vi "Find Monitor Recorders.vi"(8 "error in (no error)":errorcluster, 11 "Monitor-Pulse in":refnum<class "Monitor-Pulse.lvclass">) -> (0 "error out":errorcluster, 2 "Actot names out":string[](array[string]), 3 "Monitor-Pulse out":refnum<class "Monitor-Pulse.lvclass">)   [LabVIEW 2015, in "Monitor-Pulse.lvclass"]
uses:
  Monitor-Pulse.lvclass
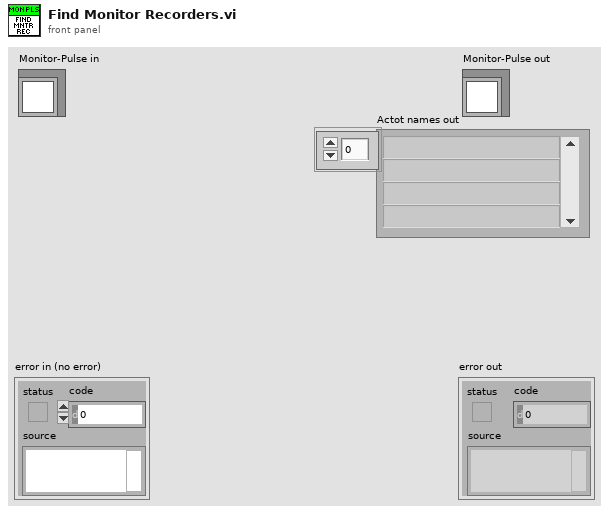
[diagram p1: front panel]
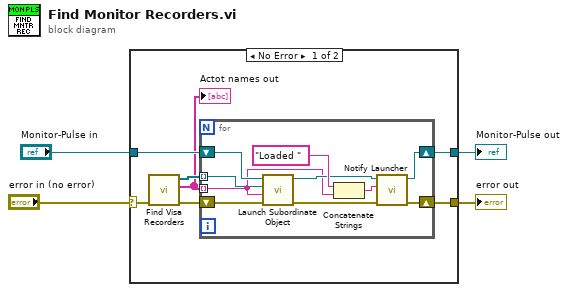
[diagram p0: block diagram]
diagram:
  n1 = case shown="No Error" "error in (no error)" {
    selector: "error in (no error)" -> [w11 w23]
    tunnel: [w7 w23] -> w3
    tunnel: [w9 w22] -> w1
    tunnel: "Monitor-Pulse in" -> [w10 w22]
    frame No Error {
      n2 = call "Find Visa Recorders.vi"("Error In"=w11) -> ("Error Out"=w8:errorcluster, "Names"=w5:string[], "Recorders List"=w6:refnum<class "Instrument Recorder.lvclass">[])  [unwired: 8 in]
      "Actot names out" <- w5
      n3 = for {
        shift-right: [w15] -> w9
        shift-left: w10 -> [w21]
        shift-right: [w13] -> w7
        shift-left: w8 -> [w20]
        tunnel: w6 -> [w19] mode=indexing
        tunnel: w5 -> [w12] mode=indexing
        n4 = call-dynamic "Launch Subordinate Object.vi"("error in (no error)"=w20, "Name"=w12, "Subordinate Object"=w19, "Measure Object in"=w21) -> ("error out"=w14:errorcluster, "Measure Object out"=w16:refnum<class "Monitor-Pulse.lvclass">)  [unwired: 5 in, 1 out]
        n5 = Concatenate Strings("Loaded " ("string"), w12) -> (w17:string)
        n6 = call-dynamic "Notify Launcher.vi"("error in (no error)"=w14, "Notification"=w17, "Measure Controller in"=w16) -> ("error out"=w13:errorcluster, "Measure Controller out"=w15:refnum<class "Monitor-Pulse.lvclass">)  [unwired: 7 in]
      }
    }
    frame Error {
    }
  }
  "error out" <- w3
  "Monitor-Pulse out" <- w1
